vi "Lcm.vi"(1 "y":i32, 2 "x":i32) -> (0 "lcm(x,y)":i64)   [LabVIEW 2018, in "NI_Gmath.lvlib"]
doc: "Computes the least common multiple of the input values."
uses:
  NI_Gmath.lvlib
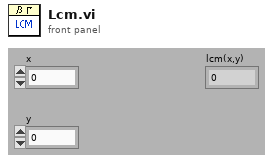
[diagram p1: front panel]
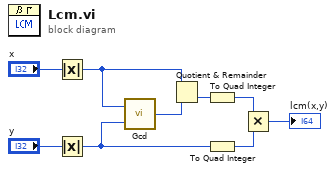
[diagram p0: block diagram]
diagram:
  n1 = Absolute Value(x="x") -> (abs(x)=w6:i32)
  n2 = Absolute Value(x="y") -> (abs(x)=w4:i32)
  n3 = call "Gcd.vi"("y"=w4, "x"=w6) -> ("gcd(x,y)"=w7:i32)
  n4 = Quotient & Remainder(x=w6, y=w7) -> (floor(x/y)=w5:i32)  [unwired: 1 out]
  n5 = To Quad Integer(1:w5) -> (0:w1:i64)
  n6 = To Quad Integer(1:w4) -> (0:w2:i64)
  n7 = Multiply(x=w1, y=w2) -> (x*y=→"lcm(x,y)":i64)
